vi "Find String in Array.vi"(9 "String":string, 10 "Array":string[](array[string])) -> (2 "Index":i32)   [LabVIEW 2020]
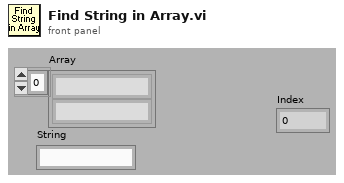
[diagram p1: front panel]
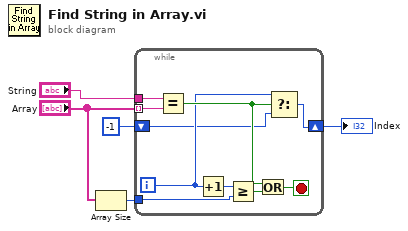
[diagram p0: block diagram]
diagram:
  n1 = Array Size(array="Array") -> (size(s)=w4:i32)
  n2 = while {
    tunnel: "Array" -> [w14] mode=indexing
    tunnel: "String" -> [w15]
    tunnel: w4 -> [w6]
    shift-right: [w8] -> w1
    shift-left: -1 ("f") -> [w9]
    i -> [w10]
    stop <- w12 stop-if-true
    n3 = Equal?(x=w15, y=w14) -> (x = y?=w11:bool)
    n4 = Increment(x=w10) -> (x+1=w7:i32)
    n5 = Greater Or Equal?(x=w7, y=w6) -> (x >= y?=w13:bool)
    n6 = Or(x=w11, y=w13) -> (x .or. y?=w12:bool)
    n7 = Select(t=w10, s=w11, f=w9) -> (s? t:f=w8:i32)
  }
  "Index" <- w1
